vi "Get Project Name.vi"(8 "error in (no error)":errorcluster, 10 "ProjectNamesIn":string[](array[string])) -> (0 "error out":errorcluster, 1 "ProjectNameOut":string, 2 "Cancel?":bool)   [LabVIEW 2019]
panel:
  in  "Project Name":string
  in  "Cancel":bool
  in  "Done":bool
  # "Please Enter Project Name"
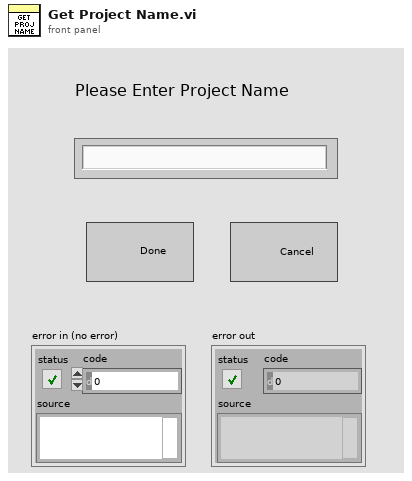
[diagram p1: front panel]
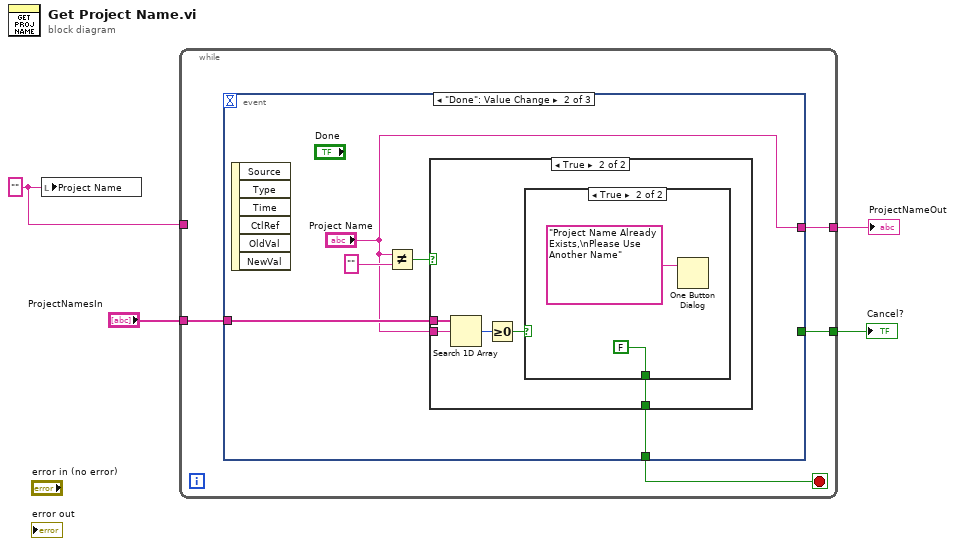
[diagram p0: block diagram]
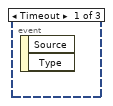
[diagram p2: hidden frame]
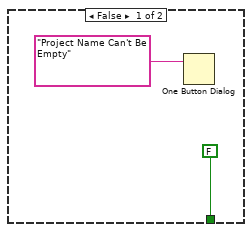
[diagram p3: hidden frame]
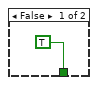
[diagram p4: hidden frame]
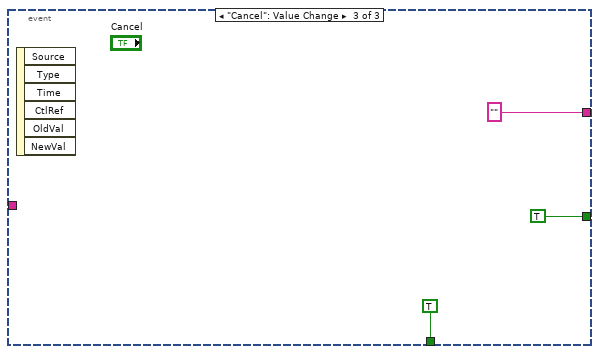
[diagram p5: hidden frame]
diagram:
  w2 = "" ("Project Name")
  n1 = local write "Project Name"(w2) -> ()
  n2 = while {
    tunnel: [w7] -> w4
    tunnel: [w6] -> w3
    tunnel: w2 -> [_]
    tunnel: "ProjectNamesIn" -> [w5]
    stop <- w8 stop-if-true
    n3 = event shown="[1] \"Done\": Value Change" {
      selector: _ -> [_ _ _]
      dyn-events: _ -> [_ _ _]
      timeout: _ -> [_ _ _]
      tunnel: [_ w11 TRUE] -> w8
      tunnel: [_ _ TRUE] -> w7
      tunnel: [_ "Project Name" "" ("Project Name")] -> w6
      tunnel: w5 -> [_ w10 _]
      event Timeout {
        n4 = event-data() -> ()  [unwired: 1 in, 2 out]
      }
      event "Done": Value Change {
        n5 = event-data() -> ()  [unwired: 1 in, 6 out]
        n6 = Not Equal?(x="Project Name", y="") -> (x != y?=w12:bool)
        n7 = case shown="True" w12 {
          tunnel: [FALSE w16] -> w11
          tunnel: w10 -> [_ w20]
          tunnel: "Project Name" -> [_ w19]
          frame False {
            n8 = One Button Dialog(message="Project Name Can't Be Empty") -> ()  [unwired: 1 in, 1 out]
          }
          frame True {
            n9 = Search 1D Array(1D array=w20, element=w19) -> (index of element=w18:i32)  [unwired: 1 in]
            n10 = Greater Or Equal To 0?(x=w18) -> (x >= 0?=w17:bool)
            n11 = case shown="True" w17 {
              tunnel: [TRUE FALSE] -> w16
              frame False {
              }
              frame True {
                n12 = One Button Dialog(message="Project Name Already Exists,\nPlease Use Another Name") -> ()  [unwired: 1 in, 1 out]
              }
            }
          }
        }
      }
      event "Cancel": Value Change {
        n13 = event-data() -> ()  [unwired: 1 in, 6 out]
      }
    }
  }
  "ProjectNameOut" <- w3
  "Cancel?" <- w4
